vi "SigMath Class - Remove from Window List.vi"(5 "error in (no error)":errorcluster, 7 "GUI VI Ref":refnum<vi>) -> (19 "error out":errorcluster)   [LabVIEW 2020, in "SigMath.lvclass"]
uses:
  SigMath.lvclass
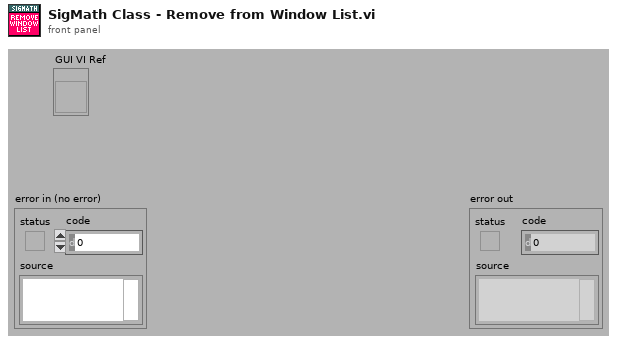
[diagram p1: front panel]
types:
  T1 = typedef "SigMath.lvclass/ClassAttributesRef.ctl" = refnum<data-value>
  T2 = typedef "SigMath.lvclass/ClassAttributes.ctl" = cluster{"Window List":refnum<vi>[]}
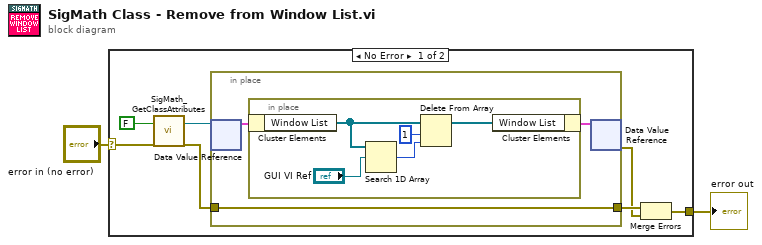
[diagram p0: block diagram]
diagram:
  n1 = case shown="No Error" "error in (no error)" {
    selector: "error in (no error)" -> [w9 w18]
    tunnel: [w6 w18] -> w1
    frame No Error {
      n2 = call "SigMath_GetClassAttributes.vi"("return data? (T)"=FALSE ("return data"), "error in (no error)"=w9) -> ("class attributes ref"=w7:T1, "error out"=w8:errorcluster)  [unwired: 14 in, 2 out]
      n3 = in-place {
        in-place-border: w8 -> [w10]
        in-place-border: [w10] -> w4
        n4 = in-place-dvr #1(w7) -> (w11:T2)  [unwired: 1 out]
        n5 = in-place {
          n6 = in-place-cluster #2(w11) -> ("Window List"=w16:refnum<vi>[])
          n7 = Search 1D Array(1D array=w16, element="GUI VI Ref") -> (index of element=w13:i32)  [unwired: 1 in]
          n8 = Delete From Array(array=w16, length=1, index=w13) -> (array with subset deleted=w15:refnum<vi>[])  [unwired: 1 out]
          n9 = in-place-cluster #2("Window List"=w15) -> (w12:T2)
        }
        n10 = in-place-dvr #1(w12) -> (w3:errorcluster)  [unwired: 1 out]
      }
      n11 = Merge Errors(w4, w3) -> (w6:errorcluster)
    }
    frame Error {
    }
  }
  "error out" <- w1
